vi "main.vi"() -> ()   [LabVIEW 2021]
uses:
  fpga/fpga_dtype_status.ctl
  core/host_global_vars.vi
panel:
  out "status":T1
  out "Server":bool
  in  "Stop server":bool
  in  "Port":u16=100
  in  "Start server":bool
  in  "Reset TG":bool
  in  "Open form":bool
  in  "Form":u16(ring) items=["feedback", "live_viewer_1D", "live_viewer_2D", "live_viewer_array", "monitor", "send_command", "slope", "xyz_monitor", "template"]
  out "command":string
  in  "Monitor avg":i32=100
  out "Command IDX":i32
  in  "Quit":bool
  in  "abort":bool
  # "OpenLabSPM"
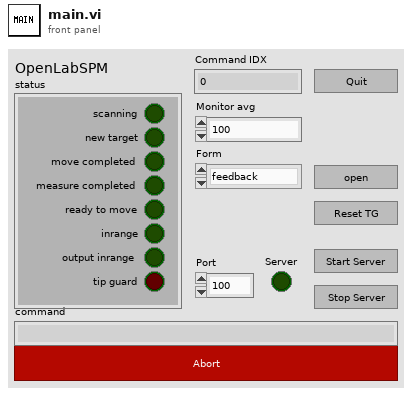
[diagram p1: front panel]
types:
  T1 = typedef "fpga_dtype_status.ctl" = cluster{"scanning":bool, "new target":bool, "move completed":bool, "measure completed":bool, "inrange":bool, "ready to move":bool, "output inrange":bool, "tip guard":bool}
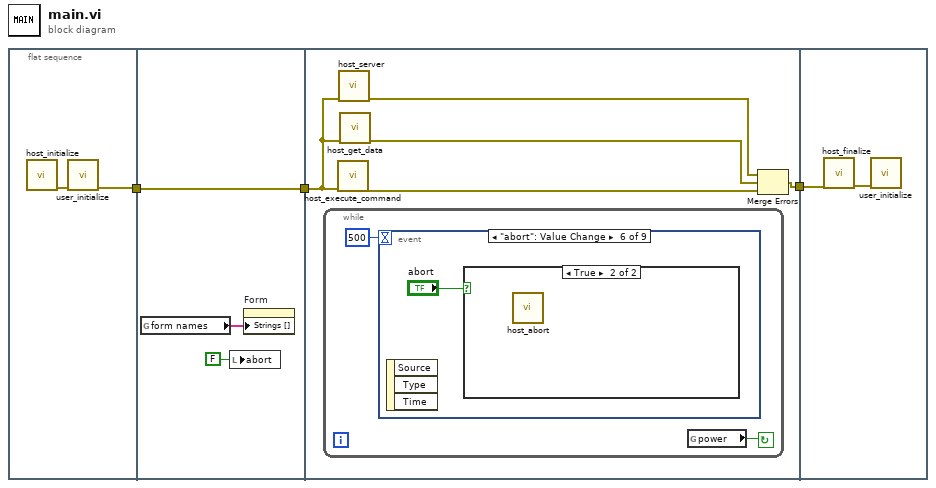
[diagram p0: block diagram]
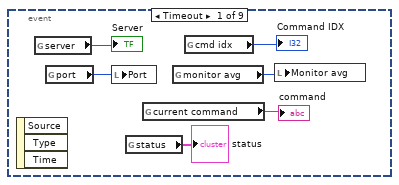
[diagram p2: hidden frame]
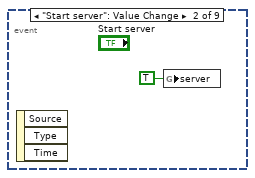
[diagram p3: hidden frame]
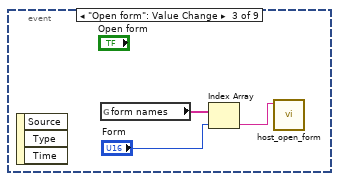
[diagram p4: hidden frame]
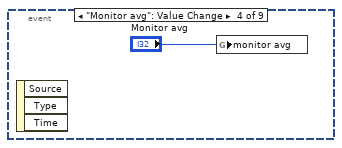
[diagram p5: hidden frame]
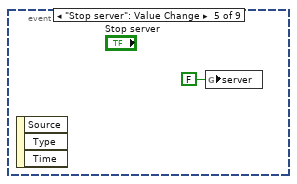
[diagram p6: hidden frame]
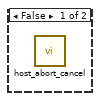
[diagram p7: hidden frame]
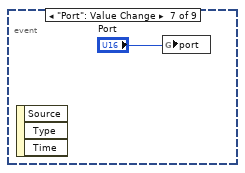
[diagram p8: hidden frame]
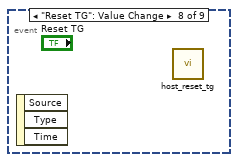
[diagram p9: hidden frame]
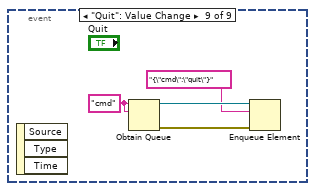
[diagram p10: hidden frame]
diagram:
  n1 = flat-sequence {
    tunnel: [w4] -> w2
    tunnel: w2 -> [w8]
    tunnel: [w8] -> w1
    tunnel: [w13] -> w3
    tunnel: w1 -> [w10]
    tunnel: w3 -> [w34]
    frame #0 {
      n2 = call "host_initialize.vi"() -> ("error out"=w5:errorcluster)  [unwired: 11 in]
      n3 = call "user_initialize.vi"("error in (no error)"=w5) -> ("error out"=w4:errorcluster)  [unwired: 10 in]
    }
    frame #1 {
      n4 = global read "host_global_vars.vi" "form names"() -> (w6:string[])
      n5 = local write "abort"(FALSE ("abort")) -> ()
      n6 = property on="Form" class="Ring (strict)"("Strings []"=w6) -> ()  [unwired: 2 in, 2 out]
    }
    frame #2 {
      n7 = while {
        stop <- w15 continue-if-true
        n8 = event shown="[5] \"abort\": Value Change" {
          selector: _ -> [_ _ _ _ _ _ _ _ _]
          dyn-events: _ -> [_ _ _ _ _ _ _ _ _]
          timeout: 500 -> [_ _ _ _ _ _ _ _ _]
          event Timeout {
            n9 = event-data() -> ()  [unwired: 1 in, 3 out]
            n10 = global read "host_global_vars.vi" "server"() -> (→"Server":bool)
            n11 = global read "host_global_vars.vi" "port"() -> (w18:u16)
            n12 = local write "Port"(w18) -> ()
            n13 = global read "host_global_vars.vi" "status"() -> (→"status":T1)
            n14 = global read "host_global_vars.vi" "current command"() -> (→"command":string)
            n15 = global read "host_global_vars.vi" "monitor avg"() -> (w20:i32)
            n16 = global read "host_global_vars.vi" "cmd idx"() -> (→"Command IDX":i32)
            n17 = local write "Monitor avg"(w20) -> ()
          }
          event "Start server": Value Change {
            n18 = event-data() -> ()  [unwired: 1 in, 3 out]
            n19 = global write "host_global_vars.vi" "server"(TRUE ("server")) -> ()
          }
          event "Open form": Value Change {
            n20 = event-data() -> ()  [unwired: 1 in, 3 out]
            n21 = global read "host_global_vars.vi" "form names"() -> (w25:string[])
            n22 = Index Array(array=w25, index="Form") -> (element=w23:string)
            n23 = call "host_open_form.vi"("name"=w23) -> ()  [unwired: 10 in, 1 out]
          }
          event "Monitor avg": Value Change {
            n24 = event-data() -> ()  [unwired: 1 in, 3 out]
            n25 = global write "host_global_vars.vi" "monitor avg"("Monitor avg") -> ()
          }
          event "Stop server": Value Change {
            n26 = event-data() -> ()  [unwired: 1 in, 3 out]
            n27 = global write "host_global_vars.vi" "server"(FALSE ("server")) -> ()
          }
          event "abort": Value Change {
            n28 = event-data() -> ()  [unwired: 1 in, 3 out]
            n29 = case shown="True" "abort" {
              frame False {
                n30 = call "host_abort_cancel.vi"() -> ()  [unwired: 11 in, 1 out]
              }
              frame True {
                n31 = call "host_abort.vi"() -> ()  [unwired: 11 in, 1 out]
              }
            }
          }
          event "Port": Value Change {
            n32 = event-data() -> ()  [unwired: 1 in, 3 out]
            n33 = global write "host_global_vars.vi" "port"("Port") -> ()
          }
          event "Reset TG": Value Change {
            n34 = event-data() -> ()  [unwired: 1 in, 3 out]
            n35 = call "host_reset_tg.vi"() -> ()  [unwired: 11 in, 1 out]
          }
          event "Quit": Value Change {
            w30 = "cmd" ("name (unnamed)")
            n36 = event-data() -> ()  [unwired: 1 in, 3 out]
            n37 = Obtain Queue(name (unnamed)=w30, element data type=w30) -> (queue out=w32:refnum<queue>, error out=w33:errorcluster)  [unwired: 3 in, 1 out]
            n38 = Enqueue Element(queue=w32, element="{\"cmd\":\"quit\"}", error in (no error)=w33) -> ()  [unwired: 1 in, 3 out]
          }
        }
        n39 = global read "host_global_vars.vi" "power"() -> (w15:bool)
      }
      n40 = call "host_execute_command.vi"("error in (no error)"=w10) -> ("error out"=w11:errorcluster)  [unwired: 10 in]
      n41 = call "host_server.vi"("error in (no error)"=w10) -> ("error out"=w9:errorcluster)  [unwired: 10 in]
      n42 = call "host_get_data.vi"("error in"=w10) -> ("error IO"=w12:errorcluster)  [unwired: 10 in]
      n43 = Merge Errors(w9, w12, w11) -> (w13:errorcluster)
    }
    frame #3 {
      n44 = call "host_finalize.vi"("error in"=w34) -> ("error out"=w35:errorcluster)  [unwired: 10 in]
      n45 = call "user_initialize.vi"("error in (no error)"=w35) -> ()  [unwired: 10 in, 1 out]
    }
  }
